vi "CMI LiB Bias Flush Buffer.vi"(8 "error in":errorcluster, 11 "VISA in":refnum<visa-resource-name>) -> (0 "error out":errorcluster, 3 "VISA out":refnum<visa-resource-name>)   [LabVIEW 2013]
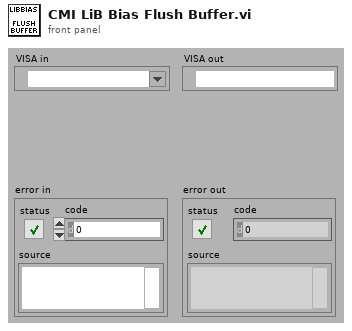
[diagram p1: front panel]
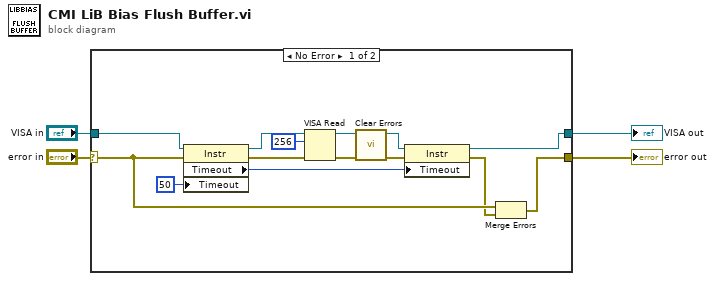
[diagram p0: block diagram]
diagram:
  n1 = case shown="No Error" "error in" {
    selector: "error in" -> [w9 w19]
    tunnel: "VISA in" -> [w16 w18]
    tunnel: [w5 w18] -> w3
    tunnel: [w7 w19] -> w2
    frame No Error {
      n2 = property class="Instr"(reference=w16, error in=w9, "Timeout"=u32 50 ("General Settings:Timeout Value")) -> (reference out=w13:refnum<visa-resource-name>, error out=w14:errorcluster, "Timeout"=w10:u32)
      n3 = VISA Read(VISA resource name=w13, byte count=u32 256, error in (no error)=w14) -> (VISA resource name out=w6:refnum<visa-resource-name>, error out=w12:errorcluster)  [unwired: 2 out]
      n4 = call <vilib>:"Clear Errors.vi"("error in (no error)"=w12) -> ("error out"=w11:errorcluster)  [unwired: 6 in]
      n5 = property class="Instr"(reference=w6, error in=w11, "Timeout"=w10) -> (reference out=w5:refnum<visa-resource-name>, error out=w8:errorcluster)
      n6 = Merge Errors(w9, w8) -> (w7:errorcluster)
    }
    frame Error {
    }
  }
  "error out" <- w2
  "VISA out" <- w3
